vi "Read DatabaseRef.vi"(8 "error in (no error)":errorcluster, 11 "Plugin in":refnum<class "Plugin.lvclass">) -> (0 "error out":errorcluster, 2 "Database.lvlib:Database":refnum<class "Database.lvclass">, 3 "Plugin out":refnum<class "Plugin.lvclass">)   [LabVIEW 2015, in "ActorManagement.lvlib" / "Plugin.lvclass"]
uses:
  Plugin.lvclass
  DatabaseManagement/Database.lvclass
  Plugin.lvclass/Plugin.ctl
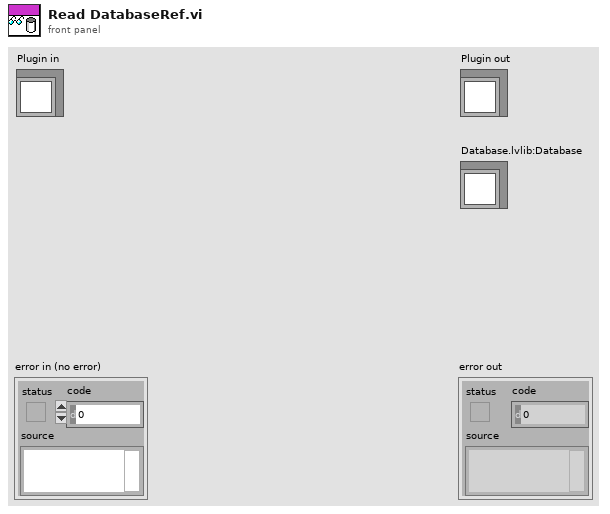
[diagram p1: front panel]
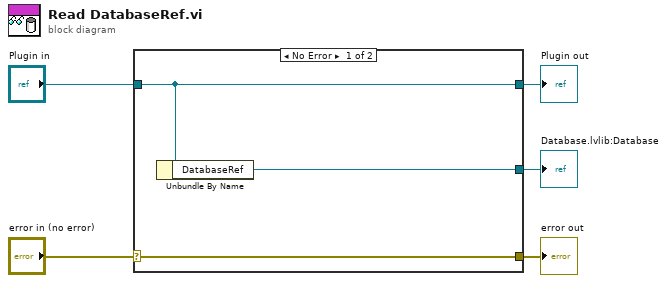
[diagram p0: block diagram]
diagram:
  n1 = case shown="No Error" "error in (no error)" {
    selector: "error in (no error)" -> [w8 w9]
    tunnel: [w8 w9] -> w4
    tunnel: [w7 w10] -> w2
    tunnel: "Plugin in" -> [w7 w10]
    tunnel: [w6 _] -> w1
    frame No Error {
      n2 = Unbundle By Name(w7) -> ("DatabaseRef"=w6:refnum<class "Database.lvclass">)
    }
    frame Error {
    }
  }
  "error out" <- w4
  "Plugin out" <- w2
  "Database.lvlib:Database" <- w1
